vi "Add VI to Owner Library or Class.vi"(6 "Virtual Folder Search Results":T1, 8 "error in":errorcluster, 9 "Insert into Virtual Folder?":bool, 10 "Reference of newly created VI":refnum<vi>, 11 "Owner Reference (Library or Class)":refnum<vi>) -> (0 "error out":errorcluster)   [LabVIEW 2022 SP3]
doc: "<add doc>"
uses:
  DFS Output (cluster).ctl
panel:
  # "Development\ncontrols/indicators useful for development and testing, but which are not outputs of the VI"
  # "Input\nInputs to the VI"
  # "Output\nOutputs of the VI"
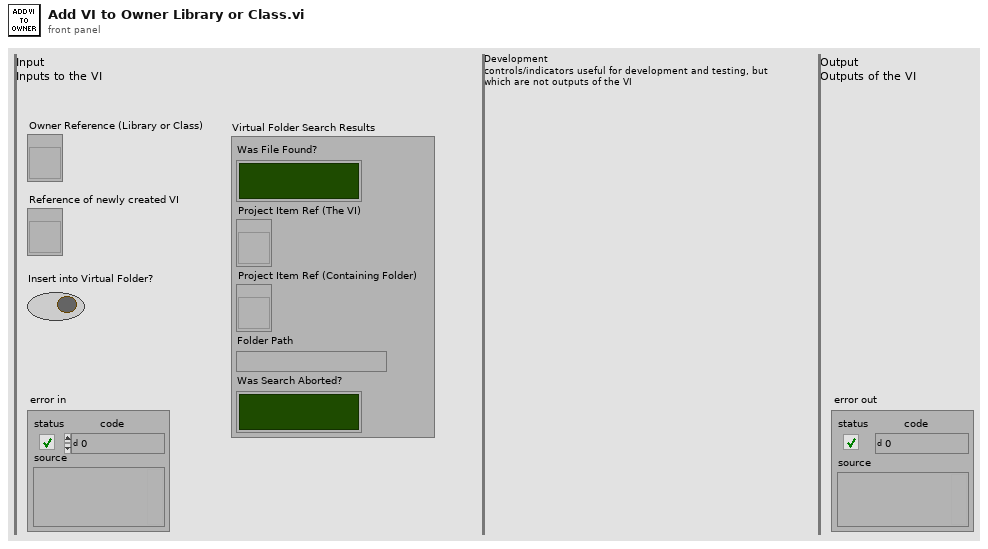
[diagram p1: front panel]
types:
  T1 = typedef "DFS Output (cluster).ctl" = cluster{"Was File Found?":bool, "Project Item Ref (The VI)":refnum<vi>, "Project Item Ref (Containing Folder)":refnum<vi>, "Folder Path":string, "Was Search Aborted?":bool}
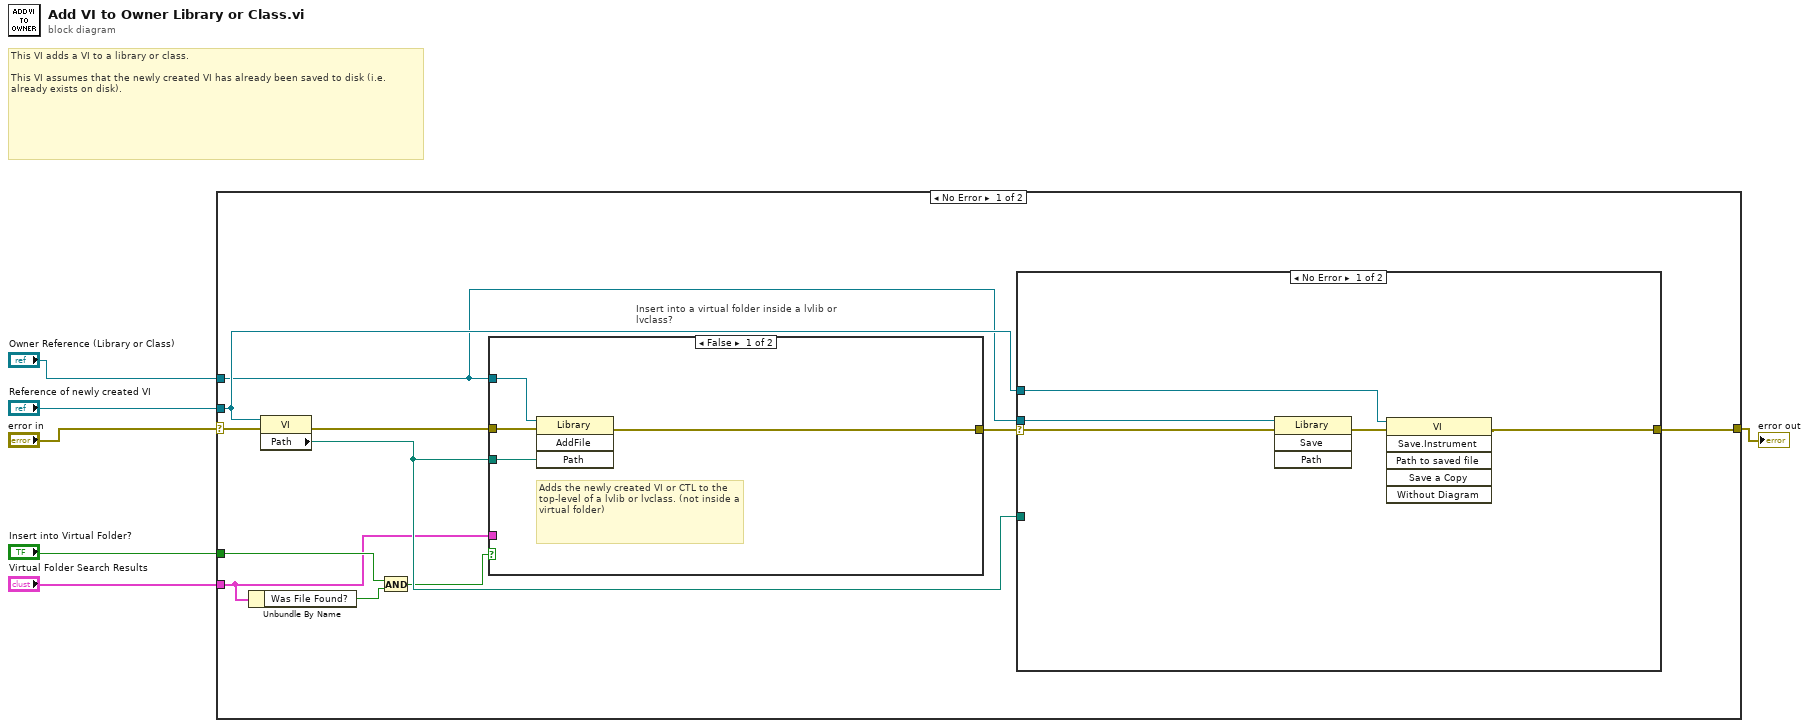
[diagram p0: block diagram]
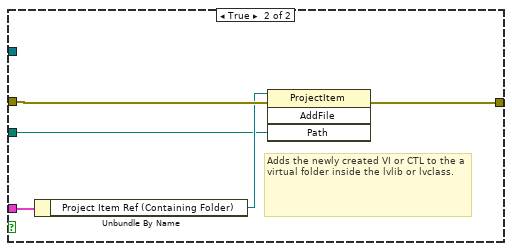
[diagram p2: hidden frame]
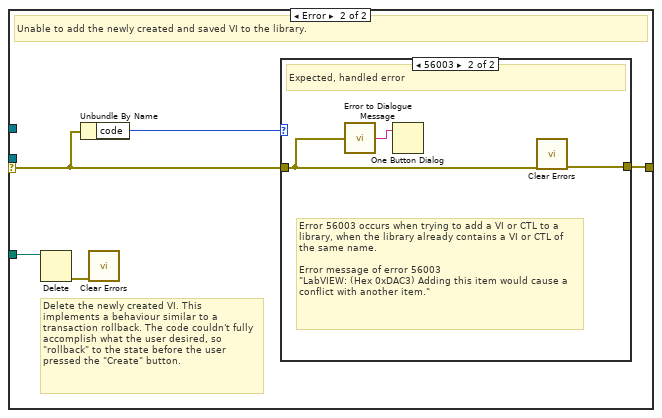
[diagram p3: hidden frame]
diagram:
  # "This VI adds a VI to a library or class.\n\nThis VI assumes that the newly created VI has already been saved to disk (i.e. already exists on disk)."
  n1 = case shown="No Error" "error in" {
    selector: "error in" -> [w17 w41]
    tunnel: [w16 w41] -> w5
    tunnel: "Owner Reference (Library or Class)" -> [w7 _]
    tunnel: "Reference of newly created VI" -> [w15 _]
    tunnel: "Virtual Folder Search Results" -> [w8 _]
    tunnel: "Insert into Virtual Folder?" -> [w14 _]
    frame No Error {
      n2 = Unbundle By Name(w8) -> ("Was File Found?"=w13:bool)
      n3 = property class="VI"(reference=w15, error in=w17) -> (error out=w11:errorcluster, "Path"=w10:path)  [unwired: 1 out]
      n4 = And(x=w14, y=w13) -> (x .and. y?=w9:bool)
      n5 = case "Insert into a virtual folder inside a lvlib or lvclass?" shown="False" w9 {
        tunnel: w7 -> [w21 _]
        tunnel: [w20 w24] -> w12
        tunnel: w11 -> [w19 w25]
        tunnel: w10 -> [w18 w22]
        tunnel: w8 -> [_ w26]
        frame False {
          # "Adds the newly created VI or CTL to the top-level of a lvlib or lvclass. (not inside a virtual folder)"
          n6 = invoke class="Library" method="AddFile"(reference=w21, error in=w19, "Path"=w18) -> (error out=w20:errorcluster)  [unwired: 1 in, 3 out]
        }
        frame True {
          # "Adds the newly created VI or CTL to the a virtual folder inside the lvlib or lvclass."
          n7 = Unbundle By Name(w26) -> ("Project Item Ref (Containing Folder)"=w23:refnum<vi>)
          n8 = invoke class="ProjectItem" method="AddFile"(reference=w23, error in=w25, "Path"=w22) -> (error out=w24:errorcluster)  [unwired: 1 in, 3 out]
        }
      }
      n9 = case shown="No Error" w12 {
        selector: w12 -> [w31 w34]
        tunnel: w7 -> [w29 _]
        tunnel: [w28 w35] -> w16
        tunnel: w15 -> [w27 _]
        tunnel: w10 -> [_ w33]
        frame No Error {
          n10 = invoke class="Library" method="Save"(reference=w29, error in=w31) -> (error out=w30:errorcluster)  [unwired: 2 in, 3 out]
          n11 = invoke class="VI" method="Save.Instrument"(reference=w27, error in=w30) -> (error out=w28:errorcluster)  [unwired: 4 in, 5 out]
        }
        frame Error {
          # "Delete the newly created VI. This implements a behaviour similar to a transaction rollback. The code couldn't fully accomplish what the user desired, so \"rollback\" to the state before the user pressed the \"Create\" button."
          # "Unable to add the newly created and saved VI to the library."
          n12 = Delete(path (use dialog)=w33) -> (error out=w32:errorcluster)  [unwired: 4 in, 2 out]
          n13 = Unbundle By Name(w34) -> ("code"=w36:i32)
          n14 = call <vilib>:"Clear Errors.vi"("error in (no error)"=w32) -> ()  [unwired: 5 in, 2 out]
          n15 = case shown="56003" w36 {
            tunnel: w34 -> [w37 w39]
            tunnel: [w37 w40] -> w35
            frame Default {
              # "Do nothing. The error will be handled downstream."
              # "Unexpected error"
            }
            frame 56003 {
              # "Error 56003 occurs when trying to add a VI or CTL to a library, when the library already contains a VI or CTL of the same name.\n\nError message of error 56003\n\"LabVIEW: (Hex 0xDAC3) Adding this item would cause a conflict with another item.\""
              # "Expected, handled error"
              n16 = call "Error to Dialogue Message.vi"("error in"=w39) -> ("Dialogue Message"=w38:string)
              n17 = One Button Dialog(message=w38) -> ()  [unwired: 1 in, 1 out]
              n18 = call <vilib>:"Clear Errors.vi"("error in (no error)"=w39) -> ("error out"=w40:errorcluster)  [unwired: 5 in, 1 out]
            }
          }
        }
      }
    }
    frame Error {
    }
  }
  "error out" <- w5
